vi "Pump Read.vi"(8 "error in (no error)":errorcluster, 9 "Message Data":variant, 11 "Hardware Resources in":T1 {"Pump Info"."Direction" items=["CW", "CCW"]; "Pump Info"."Speed" format="%03.0f"}) -> (0 "error out":errorcluster, 1 "Message Data Out":variant, 2 "Contin":bool, 3 "Hardware Resources out":T1 {"Pump Info"."Direction" items=["CW", "CCW"]; "Pump Info"."Speed" format="%03.0f"})   [LabVIEW 2020, in "Pump.lvlib"]
doc: "Perform the acquisition. Replace the contents of this diagram with calls to acquisition hardware."
uses:
  Pump.lvlib
  Pump Hardware Configuration.ctl
  support/Message Queue/Message Cluster.ctl
  support/Message Queue/Message Queue.lvlib
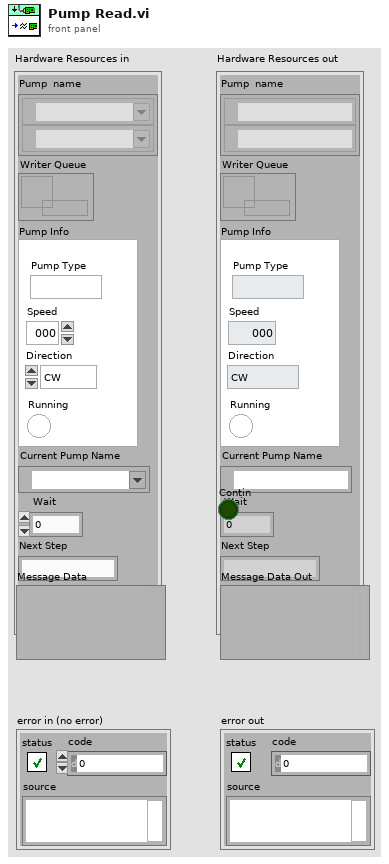
[diagram p1: front panel]
types:
  T1 = typedef "Pump.lvlib/Pump Hardware Configuration.ctl" = cluster{"Pump  name":refnum<visa-resource-name>[], "Writer Queue":refnum<queue>, "Pump Info":cluster{"Pump Type":string, "Speed":i32, "Direction":u16, "Running":bool}, "Current Pump Name":refnum<visa-resource-name>, "Wait":dbl, "Next Step":string, "Reset":bool}
  T2 = typedef "Message Queue.lvlib/Message Cluster.ctl" = cluster{"Message":string, "Message Data":variant}
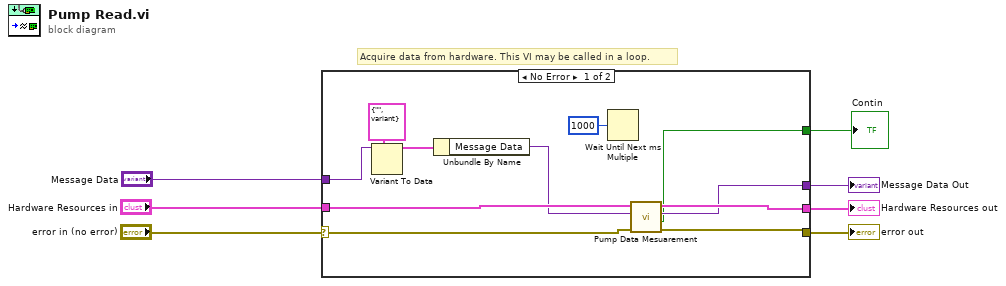
[diagram p0: block diagram]
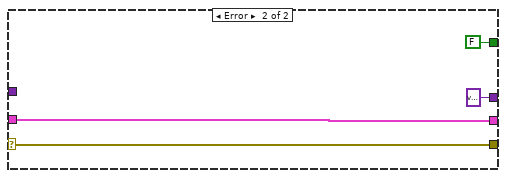
[diagram p2: hidden frame]
diagram:
  # "Acquire data from hardware. This VI may be called in a loop."
  n1 = case shown="No Error" "error in (no error)" {
    selector: "error in (no error)" -> [w18 w21]
    tunnel: [w15 w21] -> w6
    tunnel: "Hardware Resources in" -> [w17 w22]
    tunnel: [w16 w22] -> w4
    tunnel: "Message Data" -> [w10 _]
    tunnel: [w14 variant ("Message Data Out")] -> w2
    tunnel: [w9 FALSE ("Contin")] -> w1
    frame No Error {
      n2 = Variant To Data(type=T2 {"Message"="", "Message Data"=variant} ("element"), Variant=w10) -> (data=w12:T2)  [unwired: 1 in, 1 out]
      n3 = Unbundle By Name(w12) -> ("Message Data"=w11:variant)
      n4 = Wait Until Next ms Multiple(millisecond multiple=u32 1000) -> ()  [unwired: 1 out]
      n5 = call "Pump Data Mesuarement.vi"("error in (no error)"=w18, "Message Data"=w11, "Hardware Resources in"=w17) -> ("error out"=w15:errorcluster, "Contin"=w9:bool, "Message Data Out"=w14:variant, "Hardware Resources out"=w16:T1)  [unwired: 5 in]
    }
    frame Error {
    }
  }
  "Hardware Resources out" <- w4
  "error out" <- w6
  "Message Data Out" <- w2
  "Contin" <- w1
